vi "静态调用的后台任务.vi"(9 "采集速度":refnum<user-event>, 10 "采集温度":refnum<user-event>, 11 "结构名称":string="采集任务") -> (0 "错误输出":errorcluster)   [LabVIEW 2013]
uses:
  <vilib>/Platform/TimedLoop/XDataNode/timing_clust.ctl
  <vilib>/Platform/TimedLoop/XDataNode/nitl_modes.ctl
  <vilib>/Platform/TimedLoop/XDataNode/wakeup.ctl
  <vilib>/Platform/TimedLoop/XDataNode/XDataNode.xnode
  <vilib>/Platform/TimedLoop/XDataNode/XDNodeRunTimeDep.lvlib
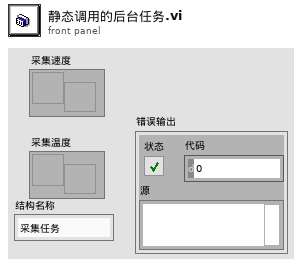
[diagram p1: front panel]
types:
  T1 = typedef "XDNodeRunTimeDep.lvlib/timing_clust.ctl" = cluster{"Expected End [f-1]":u64, "Actual End [f-1]":u64, "Finished Late? [f-1]":bool, "Expected End [i-1]":u64, "Actual End [i-1]":u64, "Finished Late? [i-1]":bool, "Expected Start [i]":u64, "Actual Start [i]":u64, "Expected Start [f]":u64, "Actual Start [f]":u64, "Source Name":string, "Structure Name":string, "Period":i64, "Deadline":i64, "Offset":i64, "Start":i64, "Priority":i32, "Timeout":i32, "Mode":T2, "Wakeup Reason":T3, "Error":errorcluster, "Source Type":string, "Secondary Source Type":string, "Global End Time":u64, "Global Start Time":u64, "Frame Duration":u64, "Iteration Duration":u64, "Assigned CPU":i32, "I/O Scan Engine Mode":u32}
  T2 = typedef "XDNodeRunTimeDep.lvlib/nitl_modes.ctl" = enum32{"No Change", "Process missed periods, maintain original phase", "Discard missed periods, maintain original phase", "Process missed periods, ignore original phase", "Discard missed periods, ignore original phase"}
  T3 = typedef "XDNodeRunTimeDep.lvlib/wakeup.ctl" = enum32{"Normal", "Aborted", "Asynchronous wakeup", "Timing source error", "Timed loop error", "Timeout"}
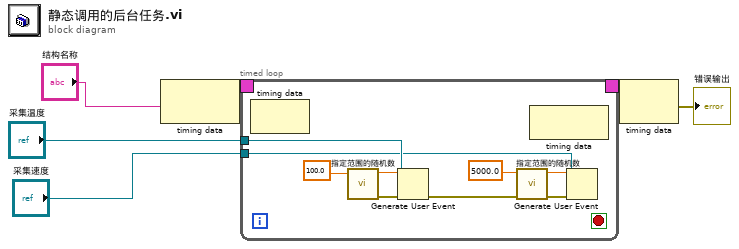
[diagram p0: block diagram]
diagram:
  n1 = node-c288("结构名称") -> (w6:T1)
  n2 = timed-loop {
    timing: w6 -> [_]
    timing-out: [_] -> w5
    tunnel: "采集温度" -> [w13]
    tunnel: "采集速度" -> [w8]
    stop <- _ stop-if-true
    n3 = node-c288() -> ()  [unwired: 1 in, 1 out]
    n4 = call-poly "指定范围的随机数.vi"("上限 (1.00)"=100.0) -> ("Error Out"=w11:errorcluster, "随机数"=w12:dbl)  [unwired: 9 in]
    n5 = Generate User Event(user event=w13, event data cluster=w12, error in=w11) -> (error out=w10:errorcluster)  [unwired: 1 in, 1 out]
    n6 = call-poly "指定范围的随机数.vi"("上限 (1.00)"=5000.0, "Error In"=w10) -> ("Error Out"=w9:errorcluster, "随机数"=w7:dbl)  [unwired: 8 in]
    n7 = node-c288() -> ()  [unwired: 1 in, 1 out]
    n8 = Generate User Event(user event=w8, event data cluster=w7, error in=w9) -> ()  [unwired: 1 in, 2 out]
  }
  n9 = node-c288(w5) -> (→"错误输出":errorcluster)
